vi "FPGA.vi"() -> ()   [LabVIEW 2023]
uses:
  <vilib>/rvi/Emulation/niFpgaGetClockAttributes.vi
  <vilib>/rvi/Emulation/niFpgaSctlEmulationGetInTimedLoop.vi
  <vilib>/rvi/Emulation/niFpgaEmulationReportErrorSimple.vi
  <vilib>/eio/utilities/niEioResolveVilibRelativePath.vi
  <vilib>/rvi/interface/RandomDataEmulation/niFpgaRandomDataHandleErrors.vi
  <vilib>/rvi/Emulation/niFpgaCriticalErrorInLSC.vi
  <vilib>/rvi/DataTransferAndStorage/Container/XNode/niFpgaContainer.xnode
  <vilib>/rvi/interface/RandomDataEmulation/nirviRandomDataFpgaReadWriteTemplate.vi
panel:
  in  "Count(uSec)":u32
  out "Actual loop rate":u32
  out "Timed Out?":bool
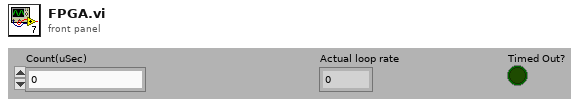
[diagram p1: front panel]
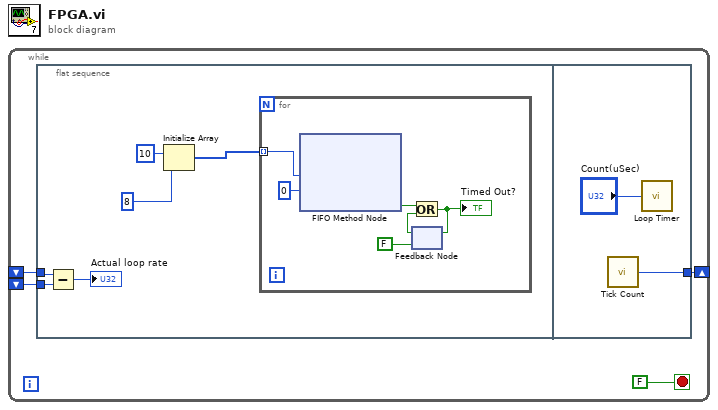
[diagram p0: block diagram]
diagram:
  n1 = while {
    shift-right: [w3] -> _
    shift-left: _ -> [w2]
    shift-left: _ -> [w1]
    stop <- FALSE stop-if-true
    n2 = flat-sequence {
      tunnel: w2 -> [w10]
      tunnel: w1 -> [w9]
      tunnel: [w18] -> w3
      frame #0 {
        n3 = Subtract(x=w10, y=w9) -> (x-y=→"Actual loop rate":u32)
        n4 = Initialize Array(i16 10 ("element"), 8 ("dimension size")) -> (w6:i16[])
        n5 = for {
          tunnel: w6 -> [w11] mode=indexing
          n6 = xnode ("FIFO Method Node")("Element"=w11, "Timeout"=0) -> ("Timed Out?"=w15:bool)  [unwired: 1 in, 1 out]
          n7 = feedback #1(FALSE) -> (w14:bool)
          n8 = Or(x=w15, y=w14) -> (x .or. y?=w13:bool)
          "Timed Out?" <- w13
          n9 = feedback-in #1(w13) -> ()
        }
      }
      frame #1 {
        n10 = call "Tick Count"() -> ("Tick Count(uSec)"=w18:u32)
        n11 = call "Loop Timer"("Count(uSec)"="Count(uSec)") -> ()  [unwired: 1 out]
      }
    }
  }
